vi "DoCalcDirection.vi"(4 "DirectionY":i8, 6 "DirectionX":i8, 8 "error in (no error)":errorcluster, 10 "SnakeGame in":refnum<class "SnakeGame.lvclass">, 11 "Snake in":refnum<class "Snake.lvclass">) -> (0 "error out":errorcluster, 1 "Direction":T1, 2 "SnakeGame out":refnum<class "SnakeGame.lvclass">, 3 "Snake out":refnum<class "Snake.lvclass">)   [LabVIEW 2019, in "RT_Game.lvlib" / "Snake.lvclass"]
uses:
  Snake.lvclass
  Direction.ctl
  SnakeGame/SnakeGame.lvclass
  Snake.lvclass/Snake.ctl
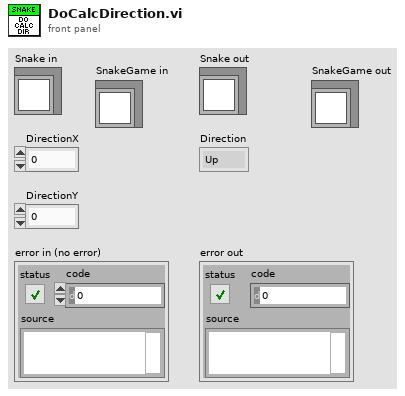
[diagram p1: front panel]
types:
  T1 = typedef "RT_Game.lvlib/Snake.lvclass/Direction.ctl" = enum16{"Up", "Left", "Down", "Right"}
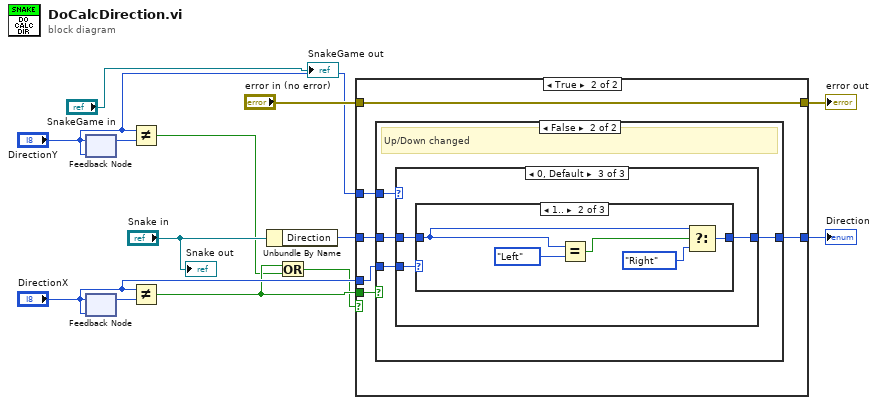
[diagram p0: block diagram]
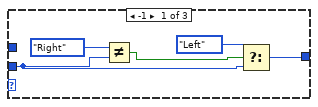
[diagram p4: hidden frame]
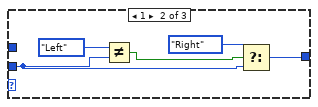
[diagram p5: hidden frame]
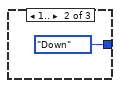
[diagram p6: hidden frame]
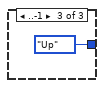
[diagram p7: hidden frame]
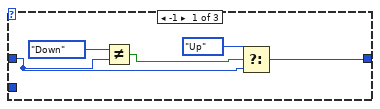
[diagram p8: hidden frame]
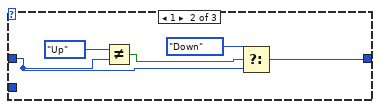
[diagram p9: hidden frame]
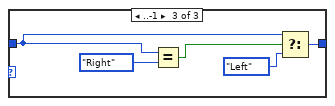
[diagram p11: hidden frame]
diagram:
  n1 = feedback #1("DirectionY") -> (w3:i8)
  n2 = feedback-in #1("DirectionY") -> ()
  n3 = feedback #2("DirectionX") -> (w2:i8)
  n4 = feedback-in #2("DirectionX") -> ()
  n5 = Not Equal?(x="DirectionY", y=w3) -> (x != y?=w4:bool)
  n6 = Not Equal?(x="DirectionX", y=w2) -> (x != y?=w6:bool)
  n7 = Unbundle By Name("Snake in") -> ("Direction"=w11:T1)
  n8 = Or(x=w6, y=w4) -> (x .or. y?=w5:bool)
  n9 = case shown="True" w5 {
    tunnel: "DirectionX" -> [_ w20]
    tunnel: "DirectionY" -> [_ w17]
    tunnel: w6 -> [_ w21]
    tunnel: w11 -> [w15 w19]
    tunnel: [w15 w18] -> w7
    tunnel: "error in (no error)" -> [w14 w16]
    tunnel: [w14 w16] -> w13
    frame False {
    }
    frame True {
      n10 = case shown="False" w21 {
        tunnel: w20 -> [w25 w42]
        tunnel: w19 -> [w24 w45]
        tunnel: [w23 w44] -> w18
        tunnel: w17 -> [w22 w43]
        frame True {
          # "Left/Right changed"
          n11 = case shown="0, Default" w25 {
            tunnel: [w28 w31 w37] -> w23
            tunnel: w24 -> [w29 w32 w36]
            tunnel: w22 -> [_ _ w38]
            frame -1 {
              n12 = Not Equal?(x=Direction."Right", y=w29) -> (x != y?=w27:bool)
              n13 = Select(t=Direction."Left", s=w27, f=w29) -> (s? t:f=w28:T1)
            }
            frame 1 {
              n14 = Not Equal?(x=Direction."Left", y=w32) -> (x != y?=w35:bool)
              n15 = Select(t=Direction."Right", s=w35, f=w32) -> (s? t:f=w31:T1)
            }
            frame 0, Default {
              n16 = case shown="0, Default" w38 {
                tunnel: [w39 Direction."Down" ("Direction") Direction."Up" ("Direction")] -> w37
                tunnel: w36 -> [w39 _ _]
                frame 0, Default {
                }
                frame 1.. {
                }
                frame ..-1 {
                }
              }
            }
          }
        }
        frame False {
          # "Up/Down changed"
          n17 = case shown="0, Default" w43 {
            tunnel: [w48 w51 w57] -> w44
            tunnel: w45 -> [w49 w52 w56]
            tunnel: w42 -> [_ _ w58]
            frame -1 {
              n18 = Not Equal?(x=Direction."Down", y=w49) -> (x != y?=w47:bool)
              n19 = Select(t=Direction."Up", s=w47, f=w49) -> (s? t:f=w48:T1)
            }
            frame 1 {
              n20 = Not Equal?(x=Direction."Up", y=w52) -> (x != y?=w55:bool)
              n21 = Select(t=Direction."Down", s=w55, f=w52) -> (s? t:f=w51:T1)
            }
            frame 0, Default {
              n22 = case shown="1.." w58 {
                tunnel: [w59 w60 w65] -> w57
                tunnel: w56 -> [w59 w62 w66]
                frame 0, Default {
                }
                frame 1.. {
                  n23 = Equal?(x=w62, y=Direction."Left") -> (x = y?=w63:bool)
                  n24 = Select(t=w62, s=w63, f=Direction."Right" ("Direction")) -> (s? t:f=w60:T1)
                }
                frame ..-1 {
                  n25 = Equal?(x=w66, y=Direction."Right") -> (x = y?=w68:bool)
                  n26 = Select(t=w66, s=w68, f=Direction."Left" ("Direction")) -> (s? t:f=w65:T1)
                }
              }
            }
          }
        }
      }
    }
  }
  "error out" <- w13
  "Direction" <- w7
  "Snake out" <- "Snake in"
  "SnakeGame out" <- "SnakeGame in"
